vi "3_inputs_or_gate.vi"(1 "z":bool, 2 "y":bool, 3 "x":bool) -> (0 "o1":bool)   [LabVIEW 2015]
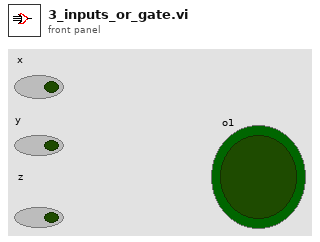
[diagram p1: front panel]
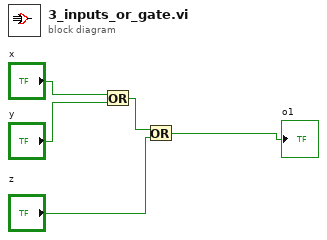
[diagram p0: block diagram]
diagram:
  n1 = Or(x="x", y="y") -> (x .or. y?=w3:bool)
  n2 = Or(x=w3, y="z") -> (x .or. y?=→"o1":bool)
